vi "Single Tone Measurement with Filtering.vi"(8 "error in (no error)":errorcluster, 10 "waveforms":waveform(dbl)[](array[waveform]), 11 "measurement configuration":T2={"digital channel list"="", "frame clock rate"=0.0, "number of channels"=0, "channel length"=0, "bit depth"=0, "data justification"=enum."Left Justified", "endianness"=enum."MSB First", "bit clock edge sync"=enum."Rising", "frame sync edge for channel 0"=enum."Rising", "channel 0 offset"=0, "master clock channel list"="", "master clock rate"=0.0, "enable dither"=FALSE, "logic level"=enum."3.3 V", "signal frequency"=1000.0, "output level"=0.0, "output level units"=enum."% FS", "output range (pk-pk)"=0.0, "load impedance"=0.0, "signal phase"=0.0, "acq sampling rate"=0.0, "min measurement cycles"=0, "min measurement time (s)"=0.0, "min settling cycles"=0, "min settling time (s)"=0.0, "acq channel"="", "band start"=0.0, "band stop"=0.0, "weighting filter"=enum."Linear", "highpass filter"=enum."DC", "lowpass filter"=enum."No filter", "SNR units"=enum."dB", "THD+N units"=enum."dB", "THD units"=enum."dB", "gain units"=enum."dB"} {"signal phase" format="%0.2f"; "master clock rate" format="%#_6pHz"; "frame clock rate" format="%#_6pHz"}) -> (0 "error out":errorcluster, 1 "spectra":cluster{"x0":dbl, "dx":dbl, "magnitude":dbl[]}[](array[cluster]), 2 "waveforms":waveform(dbl)[](array[waveform]), 3 "results":T1[](array[typedef]), 4 "output power":dbl[](array[numeric]))   [LabVIEW 2021]
uses:
  controls/single tone measurement settings (HW).ctl
  controls/digital audio protocol/data justification.ctl
  controls/digital audio protocol/endianness.ctl
  controls/digital audio protocol/digital edge.ctl
  controls/digital audio protocol/logic level.ctl
  controls/digital output level units.ctl
  controls/weighting filter.ctl
  controls/highpass filter.ctl
  controls/lowpass filter.ctl
  controls/units - snr.ctl
  controls/units - ratio.ctl
  controls/single tone audio measurements.ctl
  controls/single tone audio measurement settings.ctl
  controls/audio filter settings.ctl
  controls/units settings.ctl
  <vilib>/DAQmx/miscellaneous.llb/DAQmx Fill In Error Info.vi
  <vilib>/Waveform/WDTOps.llb/WDT Get Waveform Subset DBL.vi
  controls/audio controls.lvlib
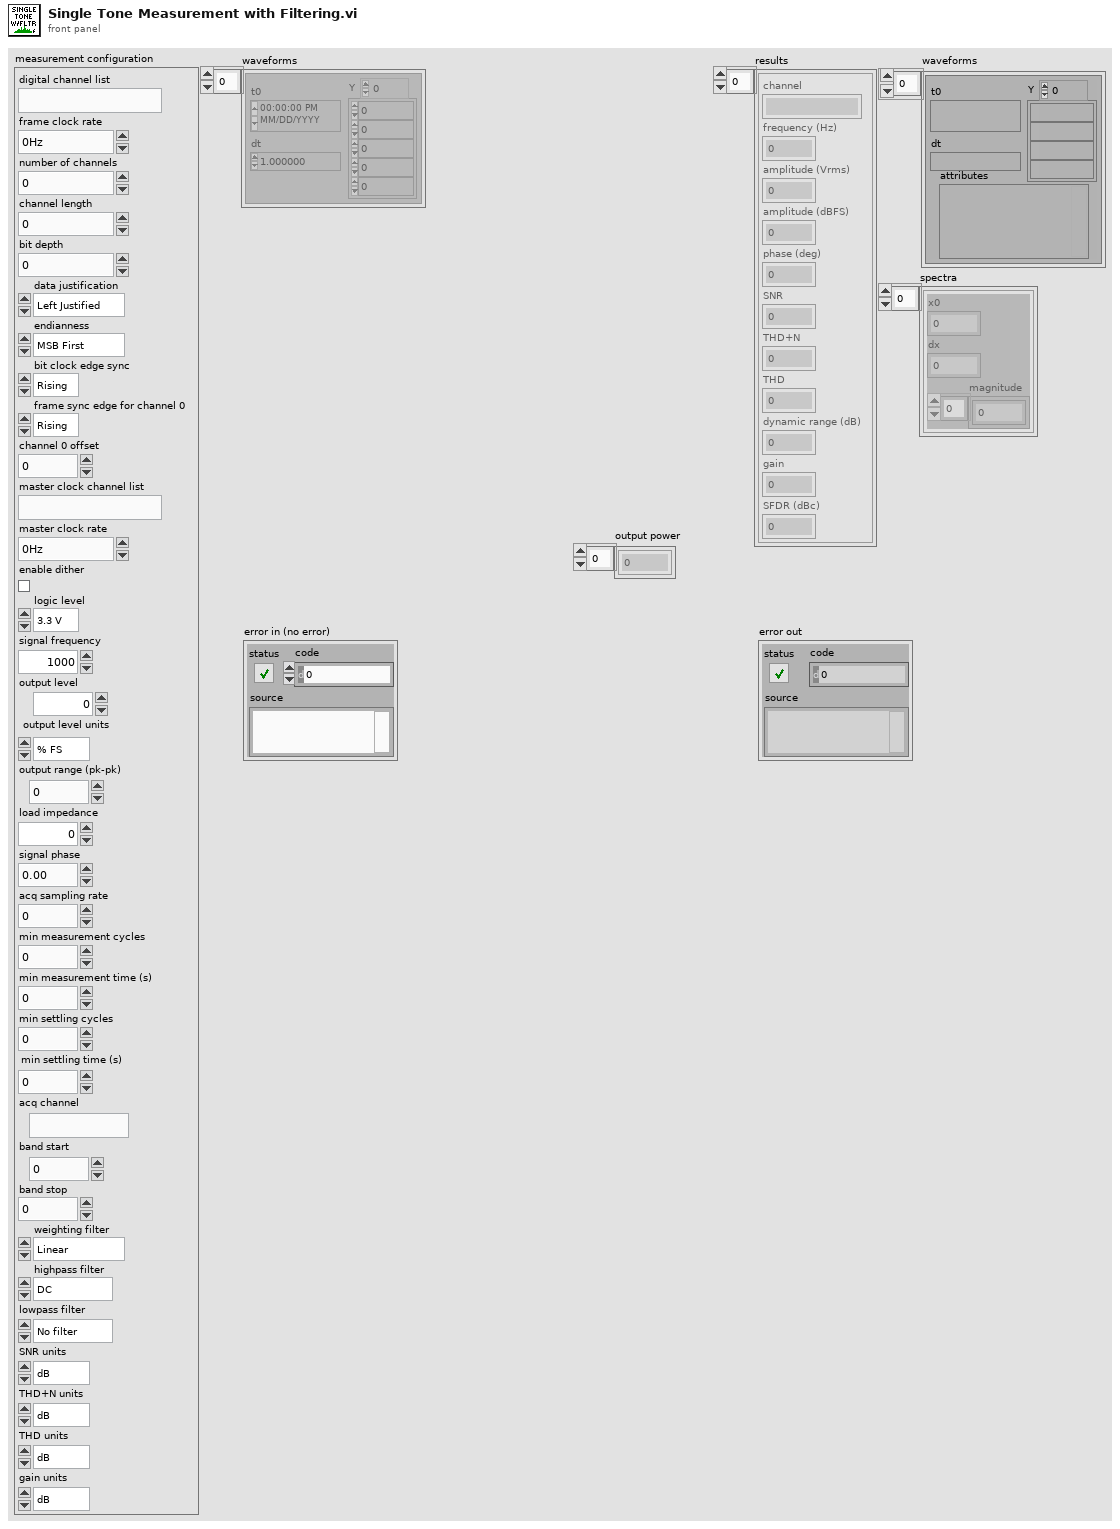
[diagram p1: front panel]
types:
  T1 = typedef "audio controls.lvlib/single tone audio measurements.ctl" = cluster{"channel":string, "frequency (Hz)":dbl, "amplitude (Vrms)":dbl, "amplitude (dBFS)":dbl, "phase (deg)":dbl, "SNR":dbl, "THD+N":dbl, "THD":dbl, "dynamic range (dB)":dbl, "gain":dbl, "SFDR (dBc)":dbl}
  T2 = typedef "single tone measurement settings (HW).ctl" = cluster{"digital channel list":string, "frame clock rate":dbl, "number of channels":u32, "channel length":u32, "bit depth":u32, "data justification":T3, "endianness":T4, "bit clock edge sync":T5, "frame sync edge for channel 0":T5, "channel 0 offset":u32, "master clock channel list":string, "master clock rate":dbl, "enable dither":bool, "logic level":T6, "signal frequency":dbl, "output level":dbl, "output level units":T7, "output range (pk-pk)":dbl, "load impedance":dbl, "signal phase":dbl, "acq sampling rate":dbl, "min measurement cycles":u32, "min measurement time (s)":dbl, "min settling cycles":u32, "min settling time (s)":dbl, "acq channel":string, "band start":dbl, "band stop":dbl, "weighting filter":T8, "highpass filter":T9, "lowpass filter":T10, "SNR units":T11, "THD+N units":T12, "THD units":T12, "gain units":T12}
  T3 = typedef "data justification.ctl" = enum32{"Left Justified", "Right Justified"}
  T4 = typedef "endianness.ctl" = enum32{"MSB First", "LSB First"}
  T5 = typedef "digital edge.ctl" = enum32{"Rising", "Falling"}
  T6 = typedef "logic level.ctl" = enum32{"3.3 V", "1.8 V", "1.2 V"}
  T7 = typedef "audio controls.lvlib/digital output level units.ctl" = enum32{"% FS", "dBFS", "V"}
  T8 = typedef "weighting filter.ctl" = enum32{"Linear", "A-weighting", "B-weighting", "C-weighting"}
  T9 = typedef "highpass filter.ctl" = enum32{"DC", "AC"}
  T10 = typedef "lowpass filter.ctl" = enum32{"No filter", "AES17 20kHz", "AES17 40kHz"}
  T11 = typedef "audio controls.lvlib/units - snr.ctl" = enum32{"dB", "x/y"}
  T12 = typedef "audio controls.lvlib/units - ratio.ctl" = enum32{"dB", "%", "x/y"}
  T13 = typedef "audio controls.lvlib/units settings.ctl" = cluster{"SNR units":T11, "THD+N units":T12, "THD units":T12, "gain units":T12}
  T14 = typedef "audio filter settings.ctl" = cluster{"weighting filter":T8, "highpass filter":T9, "lowpass filter ":T10}
  T15 = typedef "single tone audio measurement settings.ctl" = cluster{"Band start":dbl, "Band stop":dbl, "Amplitude":dbl, "Frequency":dbl, "Full scale range":dbl}
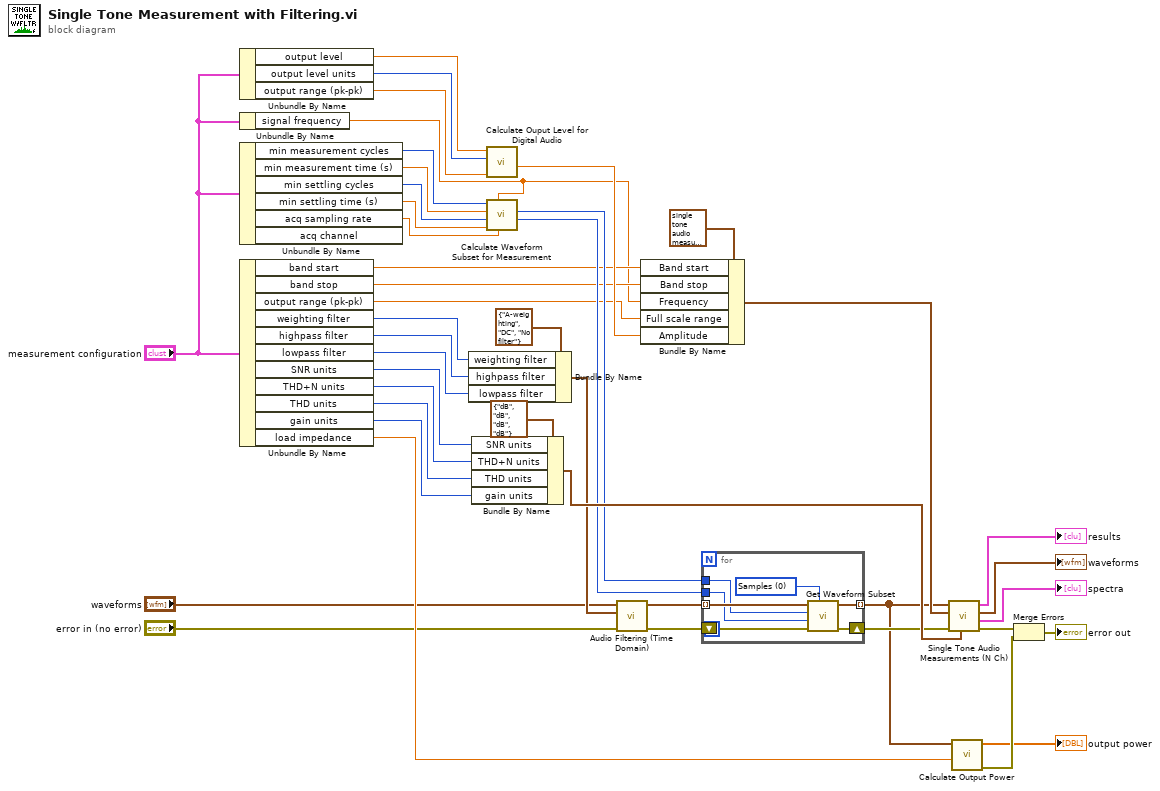
[diagram p0: block diagram]
diagram:
  n1 = Unbundle By Name("measurement configuration") -> ("output level"=w17:dbl, "output level units"=w18:T7, "output range (pk-pk)"=w19:dbl)
  n2 = Unbundle By Name("measurement configuration") -> ("signal frequency"=w9:dbl)
  n3 = Unbundle By Name("measurement configuration") -> ("min measurement cycles"=w33:u32, "min measurement time (s)"=w34:dbl, "min settling cycles"=w35:u32, "min settling time (s)"=w36:dbl, "acq sampling rate"=w27:dbl)  [unwired: 1 out]
  n4 = Unbundle By Name("measurement configuration") -> ("band start"=w12:dbl, "band stop"=w13:dbl, "output range (pk-pk)"=w16:dbl, "weighting filter"=w24:T8, "highpass filter"=w25:T9, "lowpass filter"=w26:T10, "SNR units"=w39:T11, "THD+N units"=w40:T12, "THD units"=w41:T12, "gain units"=w42:T12, "load impedance"=w43:dbl)
  n5 = Bundle By Name(cluster=T14 {"weighting filter"=enum."A-weighting", "highpass filter"=enum."DC", "lowpass filter "=enum."No filter"} ("filter settings"), "weighting filter"=w24, "highpass filter"=w25, "lowpass filter"=w26) -> (w22:T14)
  n6 = Bundle By Name(cluster=T13 {"SNR units"=enum."dB", "THD+N units"=enum."dB", "THD units"=enum."dB", "gain units"=enum."dB"} ("units settings"), "SNR units"=w39, "THD+N units"=w40, "THD units"=w41, "gain units"=w42) -> (w38:T13)
  n7 = call "Calculate Ouput Level for Digital Audio.vi"("output range (pk-pk)"=w19, "digital output level units"=w18, "output level"=w17) -> ("amplitude (pk)"=w20:dbl)  [unwired: 7 in, 1 out]
  n8 = call "Calculate Waveform Subset for Measurement.vi"("sampling rate"=w27, "signal frequency"=w9, "minimum settling duration"=w36, "minimum settling cycles"=w35, "minimum measurement duration"=w34, "minimum measurement cycles"=w33) -> ("duration (samples)"=w32:u32, "start (samples)"=w31:u32)  [unwired: 3 in, 1 out]
  n9 = call "Audio Filtering (Time Domain).vi"("waveforms"="waveforms", "filter settings"=w22, "error in"="error in (no error)") -> ("time domain"=w29:waveform(dbl)[], "error out"=w28:errorcluster)  [unwired: 6 in]
  n10 = Bundle By Name(cluster=T15 {"Band start"=20.0, "Band stop"=20000.0, "Amplitude"=-1.0, "Frequency"=1000.0, "Full scale range"=15.0} ("measurement settings"), "Band start"=w12, "Band stop"=w13, "Frequency"=w9, "Full scale range"=w16, "Amplitude"=w20) -> (w23:T15)
  n11 = for {
    tunnel: w29 -> [w50] mode=indexing
    tunnel: [w49] -> w8 mode=indexing
    shift-right: [w46] -> w30
    shift-left: w28 -> [w47]
    tunnel: w31 -> [w45]
    tunnel: w32 -> [w44]
    w48 = u16 0 items=["Samples", "Relative Time"] ("start/duration format")
    n12 = call-poly <vilib>:"Get Waveform Subset.vi"("start/duration format"=w48, "error in (no error)"=w47, "duration"=w44, "start samples/time"=w45, "waveform in"=w50) -> ("error out"=w46:errorcluster, "waveform out"=w49:waveform(dbl))  [unwired: 1 in, 2 out]
  }
  n13 = call "Single Tone Audio Measurements (N Ch).vi"("units settings"=w38, "error in"=w30, "measurement settings"=w23, "waveforms"=w8) -> ("error out"=w14:errorcluster, "spectra"=→"spectra":cluster{"x0":dbl, "dx":dbl, "magnitude":dbl[]}[], "waveforms"=→"waveforms":waveform(dbl)[], "results"=→"results":T1[])  [unwired: 4 in]
  n14 = call "Calculate Output Power.vi"("load impedance"=w43, "waveforms"=w8) -> ("error out"=w15:errorcluster, "output power"=→"output power":dbl[])  [unwired: 8 in]
  n15 = Merge Errors(w14, w15) -> (→"error out":errorcluster)
